vi "04TRM800_NextCommand.vi"(8 "error in (no error)":errorcluster, 10 "Value":i32, 11 "Enum":T1(ring)) -> (0 "error out":errorcluster, 3 "String":string)   [LabVIEW 2015]
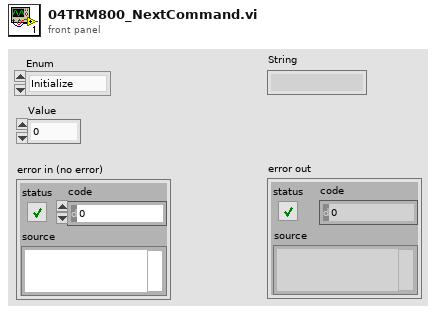
[diagram p1: front panel]
types:
  T1 = enum16{"Initialize", "Next", "SendRSET", "SetMPH", "SetINC"}
  T2 = cluster{"Pattern":enum16{"err", "mph:", "inc:", "cnfg:", "RSET"}[], "Index":i32, "mph":i32, "inc":i32}
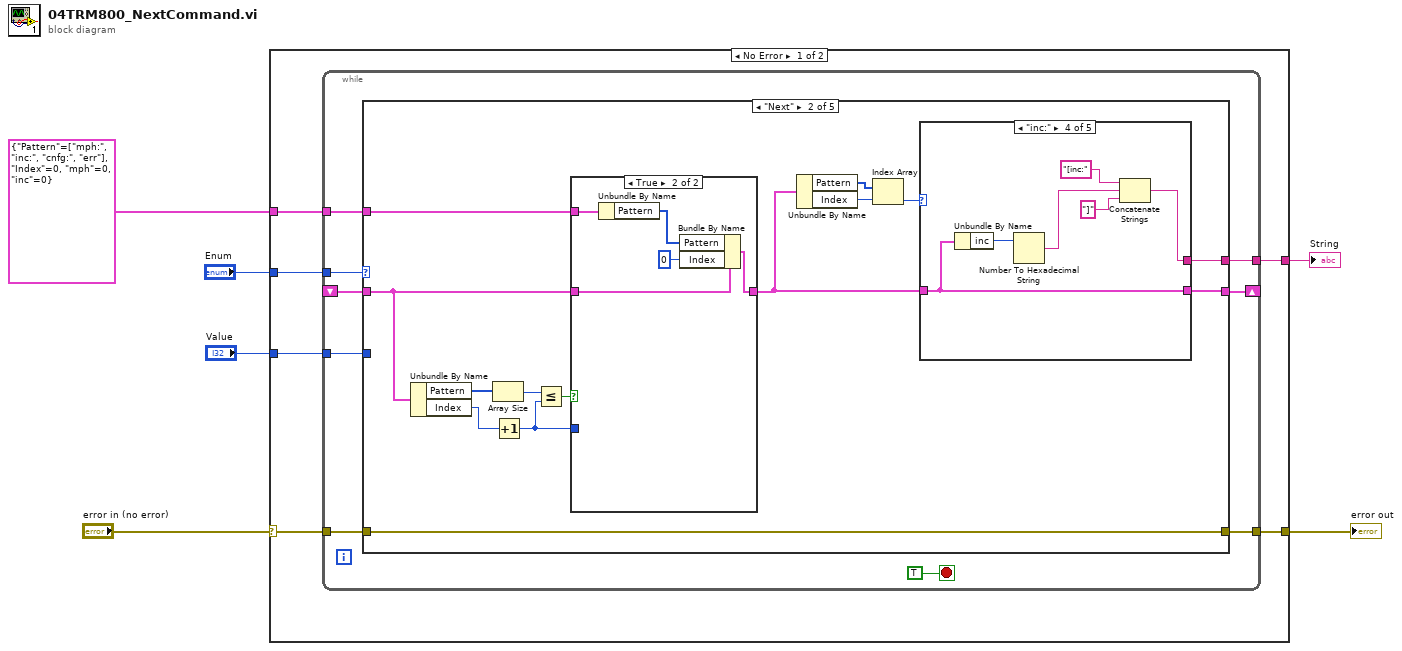
[diagram p0: block diagram]
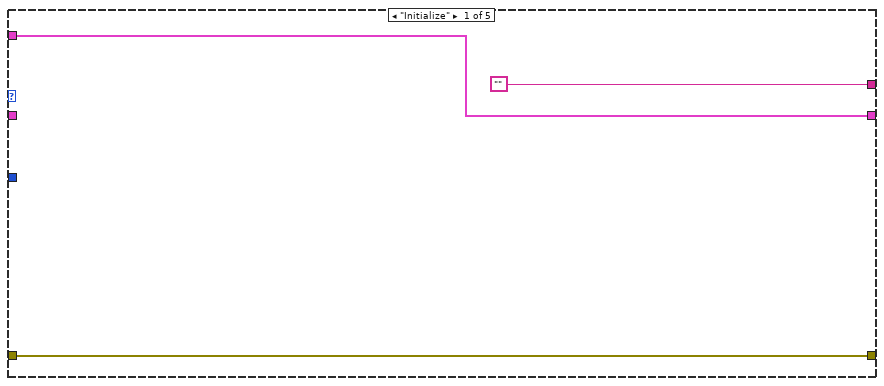
[diagram p2: hidden frame]
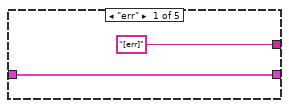
[diagram p3: hidden frame]
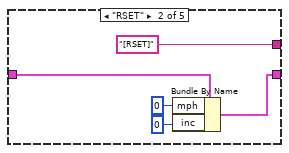
[diagram p4: hidden frame]
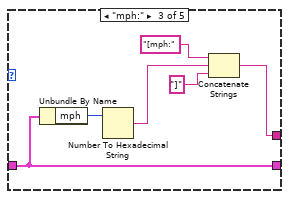
[diagram p5: hidden frame]
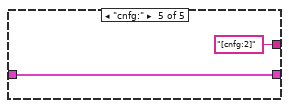
[diagram p6: hidden frame]
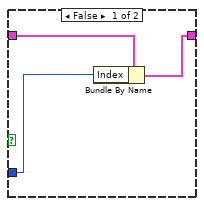
[diagram p7: hidden frame]
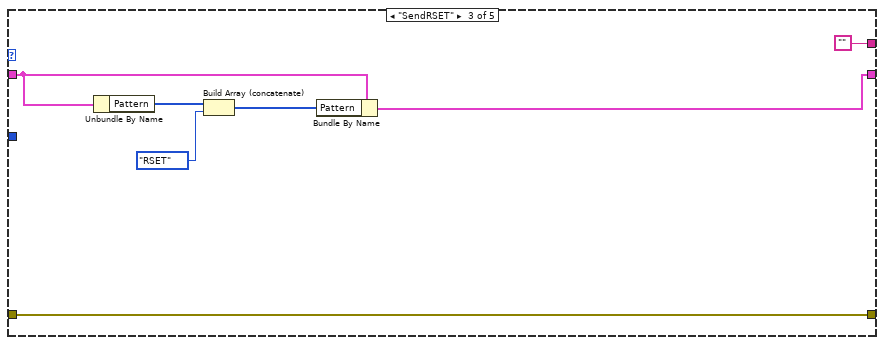
[diagram p8: hidden frame]
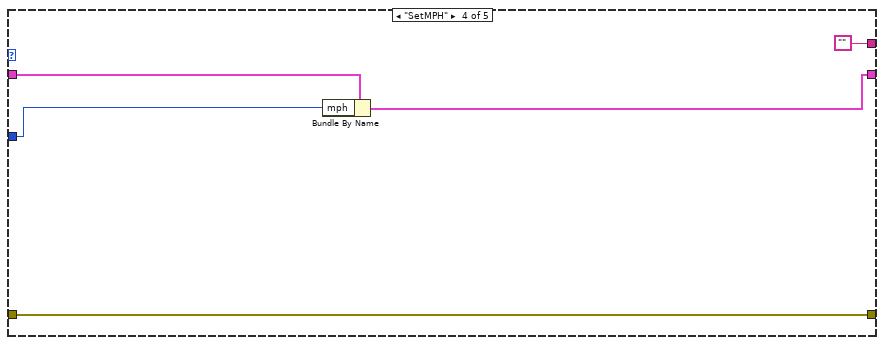
[diagram p9: hidden frame]
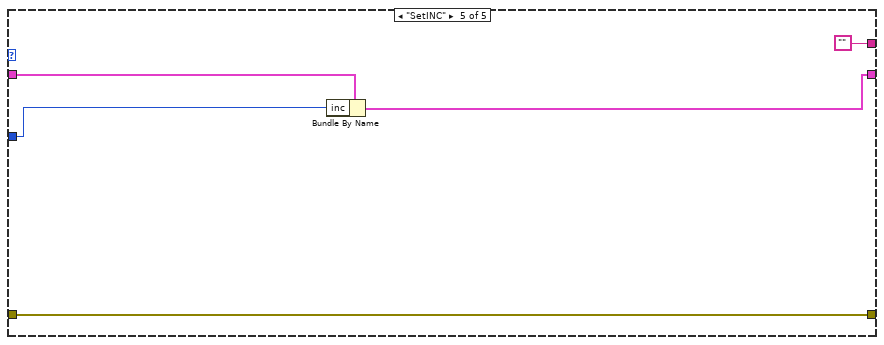
[diagram p10: hidden frame]
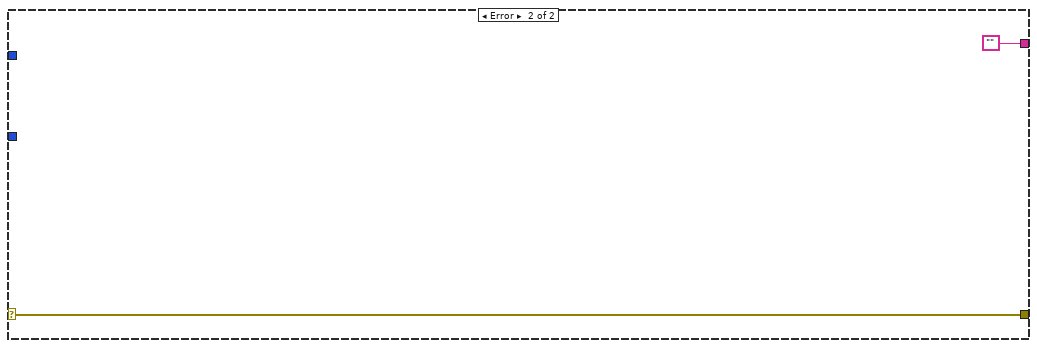
[diagram p11: hidden frame]
diagram:
  n1 = case shown="No Error" "error in (no error)" {
    selector: "error in (no error)" -> [w11 w86]
    tunnel: [w12 w86] -> w6
    tunnel: "Enum" -> [w10 _]
    tunnel: [w9 ""] -> w3
    tunnel: T2 {"Pattern"=[enum."mph:", enum."inc:", enum."cnfg:", enum."err"], "Index"=0, "mph"=0, "inc"=0} -> [w8 _]
    tunnel: "Value" -> [w7 _]
    frame No Error {
      n2 = while {
        tunnel: [w19] -> w12
        tunnel: w11 -> [w18]
        tunnel: w10 -> [w20]
        tunnel: [w17] -> w9
        tunnel: w8 -> [w16]
        shift-right: [w15] -> _
        shift-left: _ -> [w14]
        tunnel: w7 -> [w13]
        stop <- TRUE stop-if-true
        n3 = case shown="\"Next\"" w20 {
          tunnel: [w24 w38 w69 w76 w81] -> w19
          tunnel: w18 -> [w24 w38 w69 w76 w81]
          tunnel: ["" w30 "" "" ""] -> w17
          tunnel: w16 -> [w22 w34 _ _ _]
          tunnel: [w22 w25 w70 w77 w82] -> w15
          tunnel: w14 -> [_ w28 w71 w78 w83]
          tunnel: w13 -> [_ _ _ w75 w80]
          frame "Initialize" {
          }
          frame "Next" {
            n4 = Unbundle By Name(w28) -> ("Pattern"=w37:enum16{"err", "mph:", "inc:", "cnfg:", "RSET"}[], "Index"=w27:i32)
            n5 = Array Size(array=w37) -> (size(s)=w36:i32)
            n6 = Increment(x=w27) -> (x+1=w26:i32)
            n7 = Less Or Equal?(x=w36, y=w26) -> (x <= y?=w35:bool)
            n8 = case shown="True" w35 {
              tunnel: w34 -> [_ w65]
              tunnel: [w61 w66] -> w29
              tunnel: w28 -> [w62 w67]
              tunnel: w26 -> [w60 _]
              frame False {
                n9 = Bundle By Name(cluster=w62, "Index"=w60) -> (w61:T2)
              }
              frame True {
                n10 = Unbundle By Name(w65) -> ("Pattern"=w64:enum16{"err", "mph:", "inc:", "cnfg:", "RSET"}[])
                n11 = Bundle By Name(cluster=w67, "Pattern"=w64, "Index"=0) -> (w66:T2)
              }
            }
            n12 = Unbundle By Name(w29) -> ("Pattern"=w32:enum16{"err", "mph:", "inc:", "cnfg:", "RSET"}[], "Index"=w33:i32)
            n13 = Index Array(array=w32, index=w33) -> (element=w31:enum16{"err", "mph:", "inc:", "cnfg:", "RSET"})
            n14 = case shown="\"inc:\"" w31 {
              tunnel: ["[err]" "[RSET]" w50 w56 "[cnfg:2]"] -> w30
              tunnel: w29 -> [w39 w44 w46 w52 w59]
              tunnel: [w39 w43 w46 w52 w59] -> w25
              frame "err" {
              }
              frame "RSET" {
                n15 = Bundle By Name(cluster=w44, "mph"=u32 0, "inc"=u32 0) -> (w43:T2)
              }
              frame "mph:" {
                n16 = Unbundle By Name(w46) -> ("mph"=w51:i32)
                n17 = Number To Hexadecimal String(2:w51) -> (0:w49:string)  [unwired: 1 in]
                n18 = Concatenate Strings("[mph:" ("string"), w49, "]" ("string")) -> (w50:string)
              }
              frame "inc:" {
                n19 = Unbundle By Name(w52) -> ("inc"=w57:i32)
                n20 = Number To Hexadecimal String(2:w57) -> (0:w55:string)  [unwired: 1 in]
                n21 = Concatenate Strings("[inc:" ("string"), w55, "]" ("string")) -> (w56:string)
              }
              frame "cnfg:" {
              }
            }
          }
          frame "SendRSET" {
            n22 = Unbundle By Name(w71) -> ("Pattern"=w73:enum16{"err", "mph:", "inc:", "cnfg:", "RSET"}[])
            n23 = Build Array (concatenate)(w73, enum16{"err", "mph:", "inc:", "cnfg:", "RSET"}."RSET") -> (w72:enum16{"err", "mph:", "inc:", "cnfg:", "RSET"}[])
            n24 = Bundle By Name(cluster=w71, "Pattern"=w72) -> (w70:T2)
          }
          frame "SetMPH" {
            n25 = Bundle By Name(cluster=w78, "mph"=w75) -> (w77:T2)
          }
          frame "SetINC" {
            n26 = Bundle By Name(cluster=w83, "inc"=w80) -> (w82:T2)
          }
        }
      }
    }
    frame Error {
    }
  }
  "error out" <- w6
  "String" <- w3
